vi "read.vi"(1 "Index":u16, 2 "Buffer":string) -> (0 "Value":u8)   [LabVIEW 2022 SP3]
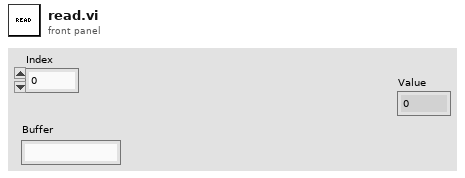
[diagram p1: front panel]
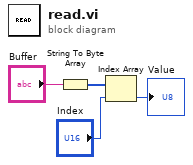
[diagram p0: block diagram]
diagram:
  n1 = String To Byte Array(string="Buffer") -> (unsigned byte array=w3:u8[])
  n2 = Index Array(array=w3, index="Index") -> (element=→"Value":u8)
